vi "Initialize Digital Edge Trigger.vi"(8 "error in (no error)":errorcluster, 11 "Digital Edge Trigger in":refnum<class "Digital Edge Trigger.lvclass">) -> (0 "error out":errorcluster, 3 "Digital Edge Trigger out":refnum<class "Digital Edge Trigger.lvclass">)   [LabVIEW 2015, in "Digital Edge Trigger.lvclass"]
uses:
  Digital Edge Trigger.lvclass
  Digital Edge Trigger.lvclass/Digital Edge Trigger.ctl
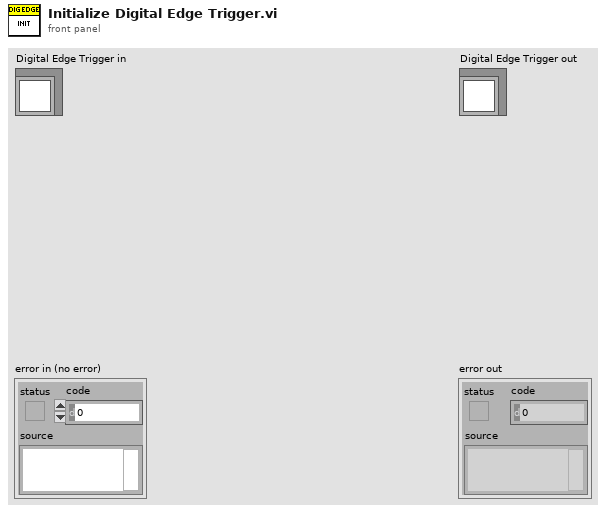
[diagram p1: front panel]
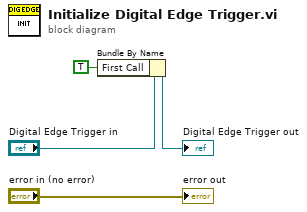
[diagram p0: block diagram]
diagram:
  n1 = Bundle By Name(cluster="Digital Edge Trigger in", "First Call"=TRUE) -> (→"Digital Edge Trigger out":refnum<class "Digital Edge Trigger.lvclass">)
  "error out" <- "error in (no error)"
